vi "Initialize sound device.vi"(2 "error in (no error)":errorcluster) -> (0 "error out":errorcluster, 1 "task ID":T1 format="%.0x")   [LabVIEW 2014]
uses:
  <vilib>/sound2/lvsound2.llb/Sound Output Task ID.ctl
  <vilib>/sound2/lvsound2.llb/Sampling Mode.ctl
  <vilib>/sound2/lvsound2.llb/Sound Data Format.ctl
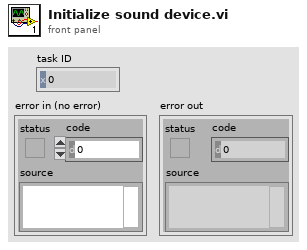
[diagram p1: front panel]
types:
  T1 = typedef "Sound Output Task ID.ctl" = u32
  T2 = typedef "Sound Data Format.ctl" = cluster{"sample rate (S/s)":dbl, "number of channels":i32, "bits per sample":i32}
  T3 = typedef "Sampling Mode.ctl" = i32
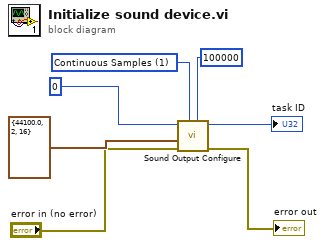
[diagram p0: block diagram]
diagram:
  w4 = T3 1 items=["Finite Samples", "Continuous Samples"] ("sample mode")
  n1 = call <vilib>:"Sound Output Configure.vi"("number of samples/ch"=100000, "sample mode"=w4, "error in (no error)"="error in (no error)", "sound format"=T2 {"sample rate (S/s)"=44100.0, "number of channels"=2, "bits per sample"=16}, "device ID"=u32 0) -> ("error out"=→"error out":errorcluster, "task ID"=→"task ID":T1)  [unwired: 5 in]
